vi "Wait on Event Sync.vi"(8 "error in (no error)":errorcluster) -> (0 "error out":errorcluster)   [LabVIEW 2016, in "CVT.lvlib"]
doc: "Wait on the rendezvous that synchronizes the registration of the events.\n_____\nBased on DQMH Project Template 6.1.0.94."
uses:
  CVT.lvlib
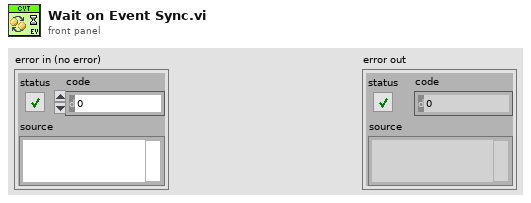
[diagram p1: front panel]
types:
  T1 = typedef "Rendezvous RefNum" = refnum<k1>
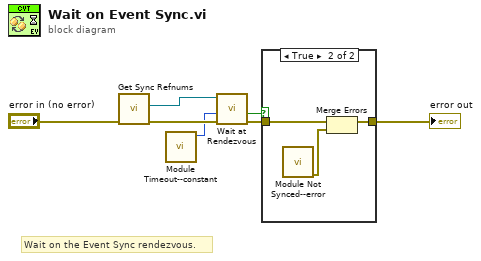
[diagram p0: block diagram]
diagram:
  # "Wait on the Event Sync rendezvous."
  n1 = call "Get Sync Refnums.vi"("error in (no error)"="error in (no error)") -> ("error out"=w6:errorcluster, "Event Sync"=w5:T1)  [unwired: 8 in, 1 out]
  n2 = call "Module Timeout--constant.vi"() -> ("Module Timeout"=w4:i32)  [unwired: 11 in]
  n3 = call <vilib>:"Wait at Rendezvous.vi"("error in (no error)"=w6, "ms timeout (-1)"=w4, "rendezvous"=w5) -> ("error out"=w2:errorcluster, "timed out"=w3:bool)  [unwired: 2 in, 1 out]
  n4 = case shown="True" w3 {
    tunnel: w2 -> [w8 w11]
    tunnel: [w8 w10] -> w1
    frame False {
    }
    frame True {
      n5 = call "Module Not Synced--error.vi"() -> ("error out"=w9:errorcluster)  [unwired: 11 in]
      n6 = Merge Errors(w11, w9) -> (w10:errorcluster)
    }
  }
  "error out" <- w1
